vi "AMQP.Test.vi"() -> ()   [LabVIEW 2016]
uses:
  <vilib>/Distrio/LabbitMQ/Connection/Connection.lvclass
  <vilib>/Distrio/LabbitMQ/Connection/connection_parameters_cluster.ctl
  global/AMQP_credentials.vi
panel:
  in  "error (in)":errorcluster
  in  "host name":string
  in  "Connection in":refnum<class "Connection.lvclass">
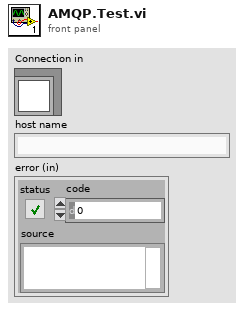
[diagram p1: front panel]
types:
  T1 = typedef "Connection.lvclass/connection_parameters_cluster.ctl" = cluster{"host name":string, "port":i32, "user name":string, "password":string, "virtual host":string}
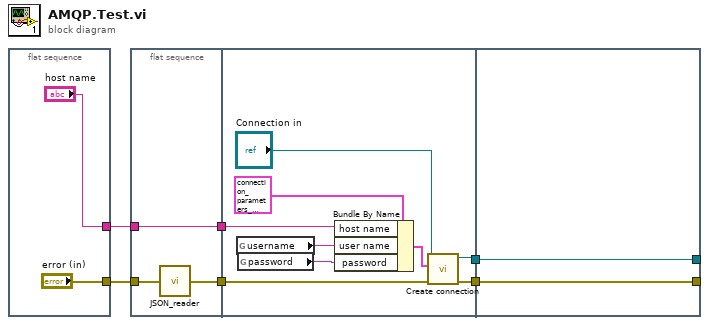
[diagram p0: block diagram]
diagram:
  n1 = flat-sequence {
    tunnel: ["error (in)"] -> w4
    tunnel: ["host name"] -> w3
    frame #0 {
    }
  }
  n2 = flat-sequence {
    tunnel: [w9] -> w6
    tunnel: [w11] -> w5
    tunnel: w4 -> [w10]
    tunnel: w3 -> [w9]
    tunnel: w6 -> [w15]
    tunnel: w5 -> [w14]
    tunnel: [w13] -> w2
    tunnel: [w12] -> w1
    tunnel: [w21] -> _
    tunnel: [w22] -> _
    tunnel: w2 -> [w22]
    tunnel: w1 -> [w21]
    frame #0 {
      n3 = call "JSON_reader.vi"("error (in)"=w10) -> ("error (out)"=w11:errorcluster)
    }
    frame #1 {
      n4 = global read "AMQP_credentials.vi" "username"() -> (w17:string)
      n5 = global read "AMQP_credentials.vi" "password"() -> (w16:string)
      n6 = Bundle By Name(cluster=T1 {"host name"="localhost", "port"=5672, "user name"="guest", "password"="guest", "virtual host"="/"} ("connection parameters"), "host name"=w15, "user name"=w17, "password"=w16) -> (w18:T1)
      n7 = call <vilib>:"Create connection.vi"("error in (no error)"=w14, "connection parameters"=w18, "Connection in"="Connection in") -> ("error out"=w12:errorcluster, "Connection out"=w13:refnum<class "Connection.lvclass">)  [unwired: 7 in]
    }
    frame #2 {
    }
  }
